vi "create event queues.vi"(11 "size":i32) -> (3 "event queue":T1)   [LabVIEW 2013, in "data bus events.lvlib"]
uses:
  data bus events.lvlib
  event queue.ctl
  event.ctl
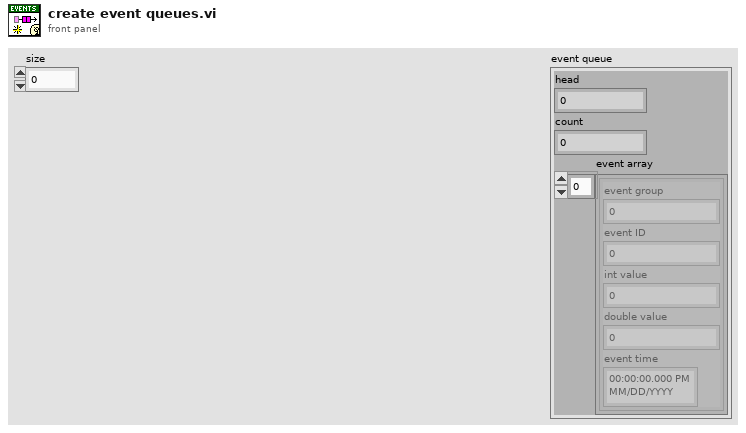
[diagram p1: front panel]
types:
  T1 = typedef "data bus events.lvlib/event queue.ctl" = cluster{"head":i32, "count":i32, "event array":T2[]}
  T2 = typedef "data bus events.lvlib/event.ctl" = cluster{"event group":i64, "event ID":i64, "int value":i64, "double value":dbl, "event time":timestamp}
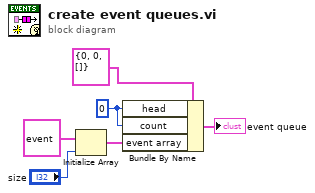
[diagram p0: block diagram]
diagram:
  w5 = 0 ("count")
  n1 = Initialize Array(T2 {"event group"=0, "event ID"=0, "int value"=0, "double value"=0.0, "event time"=timestamp(0 s since 1904-01-01)} ("event"), "size") -> (w3:T2[])
  n2 = Bundle By Name(cluster=T1 {"head"=0, "count"=0, "event array"=[]} ("event queue element"), "head"=w5, "count"=w5, "event array"=w3) -> (→"event queue":T1)
